vi "tm_getframeS16_40.vi"(7 "Options":i32(ring) items=["no option"=0, "high contrast"=16], 8 "error in (no error)":errorcluster {"code" format="%.0x"}, 10 "Frame Index":i32=-1, 11 "Handle in":u32) -> (0 "error out":errorcluster {"code" format="%.0x"}, 1 "Data B":u16[][](array[numeric]), 2 "Data A":u16[][](array[numeric]), 3 "Handle out":u32, 4 "Timestamp":dbl)   [LabVIEW 2023]
uses:
  tmcamcon.dll
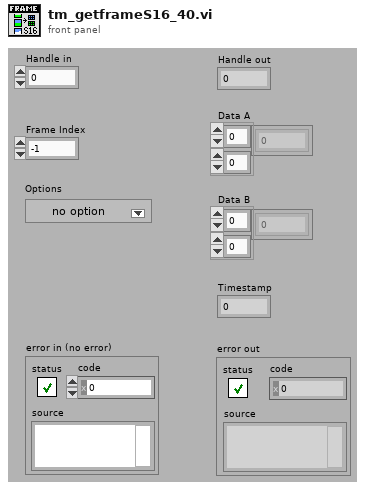
[diagram p1: front panel]
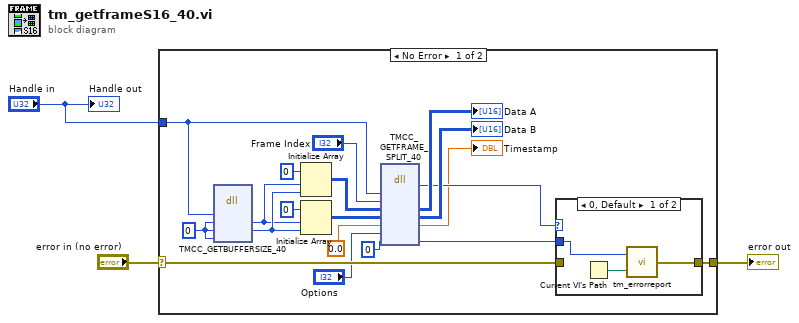
[diagram p0: block diagram]
diagram:
  n1 = case shown="No Error" "error in (no error)" {
    selector: "error in (no error)" -> [w22 w27]
    tunnel: [w21 w27] -> w2
    tunnel: "Handle in" -> [w11 _]
    frame No Error {
      w12 = 0
      n2 = dll-call lib="tmcamcon.dll" fn="TMCC_GETBUFFERSIZE_40"("index"=w11, "height"=w12, "width"=w12, "Erval"=w12) -> ("height"=w5:i32, "width"=w6:i32)  [unwired: 6 in, 2 out]
      n3 = Initialize Array(u16 0 ("element"), w5, w6) -> (w4:u16[][])
      n4 = Initialize Array(u16 0 ("element"), w5, w6) -> (w19:u16[][])
      n5 = dll-call lib="tmcamcon.dll" fn="TMCC_GETFRAME_SPLIT_40"("index"=w11, "frameindex"="Frame Index", "imgarray1"=w4, "imgarray2"=w19, "timestamp"=0.0, "option"="Options", "Erval"=0) -> ("return type"=w15:u32, "imgarray1"=→"Data A":u16[][], "imgarray2"=→"Data B":u16[][], "timestamp"=→"Timestamp":dbl, "Erval"=w14:i32)  [unwired: 6 in, 2 out]
      n6 = case shown="0, Default" w15 {
        tunnel: w22 -> [_ w26]
        tunnel: [w24 w26] -> w21
        tunnel: w14 -> [w23 _]
        frame 0, Default {
          n7 = Current VI's Path() -> (path=w25:path)
          n8 = call "tm_errorreport.vi"("Source"=w25, "Error"=w23) -> ("error out"=w24:errorcluster)
        }
        frame 1 {
        }
      }
    }
    frame Error {
    }
  }
  "error out" <- w2
  "Handle out" <- "Handle in"
